vi "Intellifaucet-Stop.vi"(0 "VISA session":refnum<visa-resource-name>="MW100", 2 "Semiphore":T1, 5 "mS wait":u32=200, 11 "Error In":errorcluster) -> (4 "dup VISA session":refnum<visa-resource-name>, 15 "Error Out":errorcluster)   [LabVIEW 2009]
uses:
  ChannelSettings.ctl
  HEWH Error Enumeration.ctl
panel:
  out "Numeric":i32
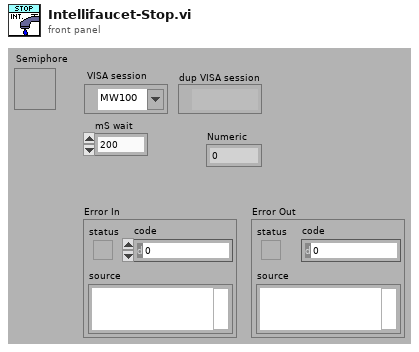
[diagram p1: front panel]
types:
  T1 = typedef "Semaphore RefNum" = refnum<k1>
  T2 = typedef "HEWH Error Enumeration.ctl" = enum16{"No Error", "GEA2 Send ACK Mismatch", "GEA2 STX", "GEA2 ETX", "GEA2 CRC Mismatch", "GEA2 ReadACK", "RTD In Range Error", "Fail Mean Tank Temp", "No Flow Config Data Found", "Failed Flow During Purge", "Temp During Purge", "Confirm IF Stop Fail", "Init Draw: TC_1 Out of Range", "Flow = 0 During Draw after 20s"}
  T3 = typedef "ChannelSettings.ctl" = u32
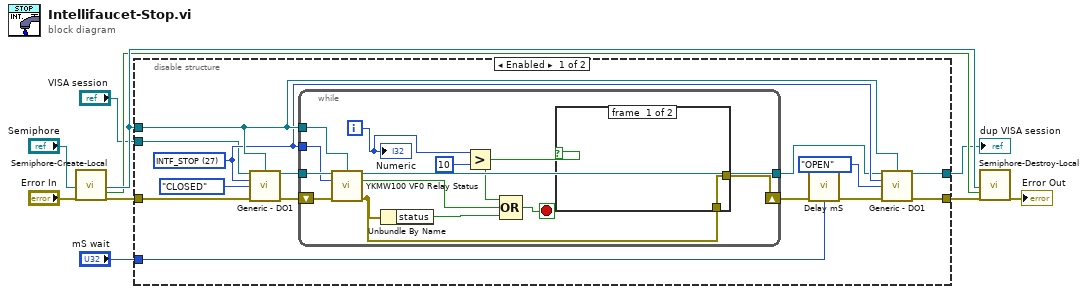
[diagram p0: block diagram]
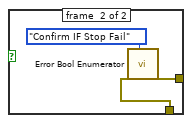
[diagram p2: hidden frame]
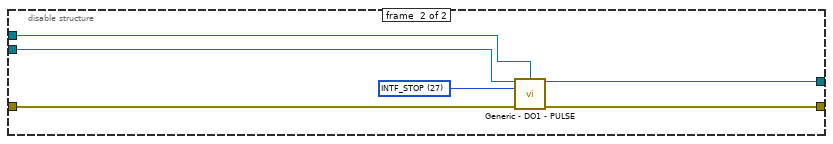
[diagram p3: hidden frame]
diagram:
  n1 = call "Semiphore-Create-Local.vi"("Semiphore"="Semiphore", "error in (no error)"="Error In") -> ("semaphore"=w8:T1, "Local?"=w7:bool, "error out"=w6:errorcluster)  [unwired: 15 in]
  n2 = disable-structure shown="Enabled" {
    disable-tunnel: [w24 w43] -> w9
    disable-tunnel: w8 -> [w23 w42]
    disable-tunnel: w6 -> [w22 w44]
    disable-tunnel: "VISA session" -> [w16 w46]
    disable-tunnel: "mS wait" -> [w12 _]
    disable-tunnel: [w11 w41] -> w1
    frame #0 {
      w21 = T3 27 items=["4-20_OUT", "Pres_HI1", "Pres_HI2", "Pres_LOW", "Pres_PIN", "HEATER_TOP", "HEATER_BOT", "T_Shell", "FLOWMETER", "WATT_SENSE", "WH_TICK", "Tc_1", "Tc_2", "Tc_3", "Tc_4", "Tc_5", "Tc_6", "Tc_down", "T_Shell_2", "T_Shell_3", "T_Shell_4", "RTD_IN", "RTD_OUT", "RTD_AMB", "INTF_TEMPFLO", "INTF_READY", "INTF_START", "INTF_STOP", "DRM_LOW", "DRM_HIGH", "PWR_MAIN", "VLV_DUMP", "VLV_OUT", "VLV_IN", "WATT_HOURS", "FLOW(SAMPLE)", "GALLONS", "FLOW(GPM)"] ("Channel_Enum")
      n3 = call "Generic - DO1.vi"("VISA session"=w16, "Semiphore"=w23, "Channel_Enum"=w21, "Relay Status (0:CLOSED)"=enum8{"CLOSED", "OPEN"}."CLOSED", "Error In"=w22) -> ("dup VISA session"=w18:refnum<visa-resource-name>, "error out"=w17:errorcluster)  [unwired: 9 in]
      n4 = while {
        tunnel: w18 -> [w37]
        tunnel: w23 -> [w36]
        tunnel: [w35] -> w20
        shift-right: [w27] -> w19
        shift-left: w17 -> [w33]
        tunnel: w21 -> [w34]
        i -> [w30]
        stop <- w31 stop-if-true
        n5 = call "YKMW100 VF0 Relay Status.vi"("VISA session"=w37, "Semiphore"=w36, "Channel_Enum"=w34, "error in (no error)"=w33) -> ("dup VISA session"=w35:refnum<visa-resource-name>, "Output On"=w25:bool, "error out"=w26:errorcluster)  [unwired: 8 in, 1 out]
        n6 = Unbundle By Name(w26) -> ("status"=w32:bool)
        n7 = Greater?(x=w30, y=10) -> (0:w28:bool)
        n8 = Compound Arithmetic op=OR(w28, w25, w32) -> (w31:bool)
        n9 = case shown="True" w28 {
          tunnel: [w38 w39] -> w27
          tunnel: w26 -> [w38 w39]
          frame #0 {
          }
          frame #1 {
            n10 = call "Error Bool Enumerator.vi"("Error Enum"=HEWH_Error_Enumeration."Confirm IF Stop Fail") -> ()  [unwired: 8 in, 1 out]
          }
        }
        "Numeric" <- w30
      }
      n11 = call "Delay mS.vi"("Error In"=w19, "milliseconds to wait"=w12) -> ("Error Out"=w13:errorcluster)  [unwired: 13 in]
      n12 = call "Generic - DO1.vi"("VISA session"=w20, "Semiphore"=w23, "Channel_Enum"=w21, "Relay Status (0:CLOSED)"=enum8{"CLOSED", "OPEN"}."OPEN", "Error In"=w13) -> ("dup VISA session"=w11:refnum<visa-resource-name>, "error out"=w24:errorcluster)  [unwired: 9 in]
    }
    frame #1 {
      w45 = T3 27 items=["4-20_OUT", "Pres_HI1", "Pres_HI2", "Pres_LOW", "Pres_PIN", "HEATER_TOP", "HEATER_BOT", "T_Shell", "FLOWMETER", "WATT_SENSE", "WH_TICK", "Tc_1", "Tc_2", "Tc_3", "Tc_4", "Tc_5", "Tc_6", "Tc_down", "T_Shell_2", "T_Shell_3", "T_Shell_4", "RTD_IN", "RTD_OUT", "RTD_AMB", "INTF_TEMPFLO", "INTF_READY", "INTF_START", "INTF_STOP", "DRM_LOW", "DRM_HIGH", "PWR_MAIN", "VLV_DUMP", "VLV_OUT", "VLV_IN", "WATT_HOURS", "FLOW(SAMPLE)", "GALLONS", "FLOW(GPM)"] ("Channel_Enum")
      n13 = call "Generic - DO1 - PULSE.vi"("VISA session"=w46, "Semiphore"=w42, "Channel_Enum"=w45, "Error In"=w44) -> ("dup VISA session"=w41:refnum<visa-resource-name>, "error out"=w43:errorcluster)  [unwired: 10 in]
    }
  }
  "dup VISA session" <- w1
  n14 = call "Semiphore-Destroy-Local.vi"("Semiphore"=w8, "Local?"=w7, "error in (no error)"=w9) -> ("error out"=→"Error Out":errorcluster)  [unwired: 16 in]
